vi "NonRedundantSwap.vi"(8 "error in (no error)":errorcluster, 10 "Schedule in":u16[](array[numeric]), 11 "OSSP_Problem in":refnum<class "OSSP_Problem.lvclass">) -> (0 "error out":errorcluster, 2 "Schedule out":u16[](array[numeric]), 3 "OSSP_Problem out":refnum<class "OSSP_Problem.lvclass">)   [LabVIEW 2013, in "GA.lvclass"]
uses:
  GA.lvclass
  OSSP_Problem.lvclass
  OSSP_Problem.lvclass/OSSP_Problem.ctl
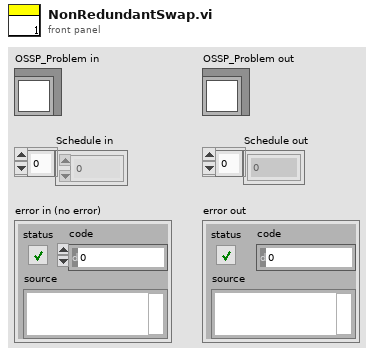
[diagram p1: front panel]
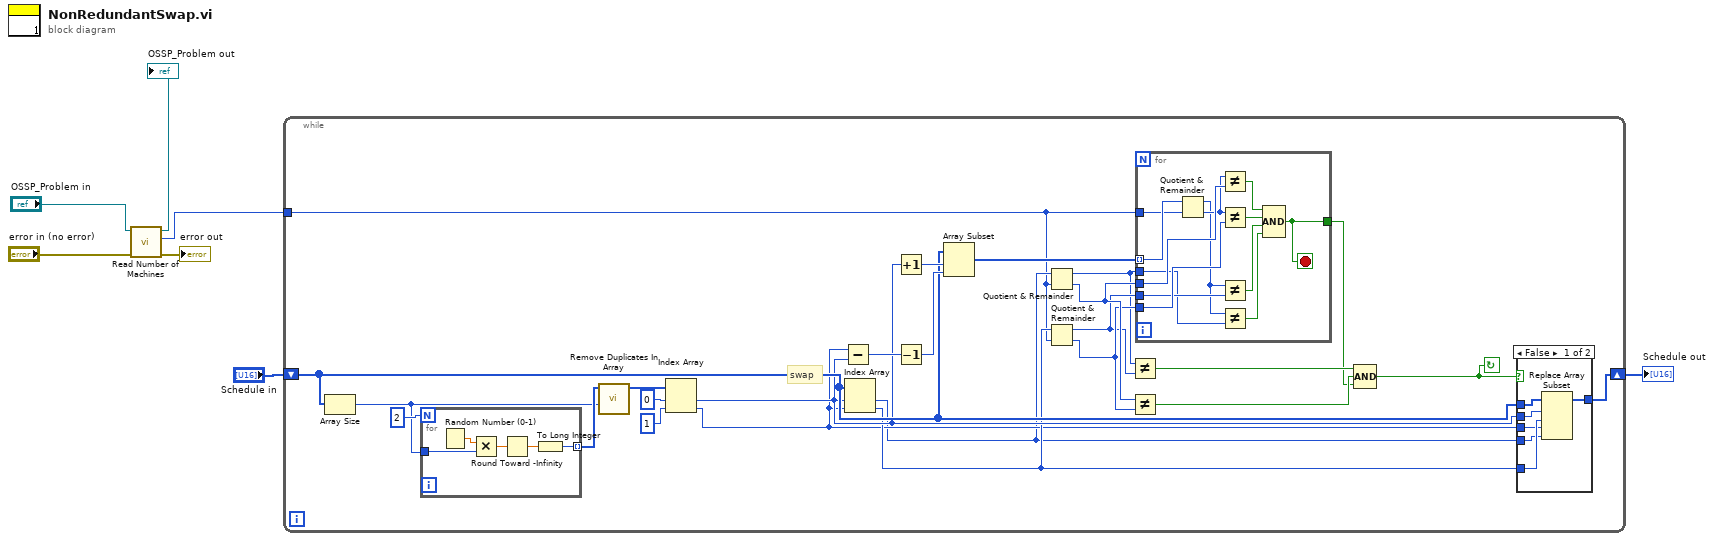
[diagram p0: block diagram]
diagram:
  n1 = call "Read Number of Machines.vi"("error in (no error)"="error in (no error)", "OSSP_Problem in"="OSSP_Problem in") -> ("error out"=→"error out":errorcluster, "Number of Machines"=w3:i32, "OSSP_Problem out"=→"OSSP_Problem out":refnum<class "OSSP_Problem.lvclass">)  [unwired: 7 in]
  n2 = while {
    shift-right: [w16] -> w2
    shift-left: "Schedule in" -> [w17]
    tunnel: w3 -> [w11]
    stop <- w18 continue-if-true
    # "swap"
    n3 = Array Size(array=w17) -> (size(s)=w9:i32)
    n4 = for {
      N: 2 -> [_]
      tunnel: w9 -> [w54]
      tunnel: [w53] -> w10 mode=indexing
      n5 = Random Number (0-1)() -> (number: 0 to 1=w57:dbl)
      n6 = Multiply(x=w57, y=w54) -> (x*y=w56:dbl)
      n7 = Round Toward -Infinity(1:w56) -> (0:w55:dbl)
      n8 = To Long Integer(number=w55) -> (32bit integer=w53:i32)
    }
    n9 = call "Remove Duplicates In Array.vi"("Max Index Bound"=w9, "Random Numbers Array"=w10) -> ("Random Numbers Array without Duplicates"=w8:i32[])  [unwired: 9 in]
    n10 = Index Array(array=w8, index #1=0 ("index"), index #2=1 ("index")) -> (element #1=w15:i32, element #2=w13:i32)
    n11 = Subtract(x=w13, y=w15) -> (x-y=w26:i32)
    n12 = Index Array(array=w17, index #1=w15, index #2=w13) -> (element #1=w12:u16, element #2=w14:u16)
    n13 = Increment(x=w15) -> (x+1=w27:i32)
    n14 = Decrement(x=w26) -> (x-1=w25:i32)
    n15 = Array Subset(array=w17, index=w27, length=w25) -> (w24:u16[])
    n16 = Quotient & Remainder(x=w12, y=w11) -> (x-y*floor(x/y)=w20:i32, floor(x/y)=w23:i32)
    n17 = Quotient & Remainder(x=w14, y=w11) -> (x-y*floor(x/y)=w21:i32, floor(x/y)=w22:i32)
    n18 = Not Equal?(x=w20, y=w21) -> (x != y?=w32:bool)
    n19 = Not Equal?(x=w23, y=w22) -> (x != y?=w31:bool)
    n20 = for {
      tunnel: w24 -> [w52] mode=indexing
      tunnel: w11 -> [w51]
      tunnel: w23 -> [w50]
      tunnel: w22 -> [w49]
      tunnel: w21 -> [w47]
      tunnel: w20 -> [w46]
      tunnel: [w40] -> w19
      stop <- w40 stop-if-true
      n21 = Quotient & Remainder(x=w52, y=w51) -> (x-y*floor(x/y)=w45:i32, floor(x/y)=w48:i32)
      n22 = Not Equal?(x=w48, y=w50) -> (x != y?=w44:bool)
      n23 = Not Equal?(x=w48, y=w49) -> (x != y?=w43:bool)
      n24 = Not Equal?(x=w45, y=w47) -> (x != y?=w42:bool)
      n25 = Not Equal?(x=w45, y=w46) -> (x != y?=w41:bool)
      n26 = Compound Arithmetic op=AND(w44, w43, w42, w41) -> (w40:bool)
    }
    n27 = Compound Arithmetic op=AND(w32, w31, w19) -> (w18:bool)
    n28 = case shown="False" w18 {
      tunnel: w17 -> [w38 w39]
      tunnel: [w33 w39] -> w16
      tunnel: w15 -> [w37 _]
      tunnel: w14 -> [w36 _]
      tunnel: w13 -> [w35 _]
      tunnel: w12 -> [w34 _]
      frame False {
        n29 = Replace Array Subset(array=w38, new element #1=w36, index #1=w37, new element #2=w34, index #2=w35) -> (w33:u16[])
      }
      frame True {
      }
    }
  }
  "Schedule out" <- w2
